vi "CreateTempSensorParam332.vi"(0 "Courbe Conv":string[](array[string]) caption="Courbe Conversion", 11 "Error in":errorcluster) -> (4 "Configurations":string[](array[string]), 6 "SavedOK":bool, 8 "ModèleSauv":i32, 15 "Error out":errorcluster)   [LabVIEW 2010]
doc: "Ce Vi sert à la création de modèles de configuration. À partir des différents paramètres d'entreés disponible, il crée une table qui constitue le modèle. Le VI permet la sauvegarde des nouveaux modèles et la gestion des modèles existant."
uses:
  <vilib>/Utility/error.llb/DialogType.ctl
  <vilib>/Utility/config.llb/NI_LVConfig.lvlib
panel:
  in  "SensorPar":T1={"TableTC"=0, "TableConv"=0, "Compensation"=1, "Type"=1} caption="Paramètre de configuration d'entrée" {"Compensation" items=["Off", "On"]; "Type" items=["Silicon Diode", "GaAlAs Diode", "Platinum 100 (250 Ohms)", "Platinum 100 (500 Ohms)", "Platinum 1000 Ohms", "NTC RTD 75mV 7.5 KOhms", "Thermocouple 25mV", "Thermocouple 50mV", "NTC RTD 75mV 75 Ohms", "NTC RTD 75mV 750 Ohms", "NTC RTD 75mV 7.5 KOhms", "NTC RTD 75mV 75 KOhms", "NTC RTD 75mV Auto"]; "TableTC" max=41 step=1}
  in  "Nom":string
  in  "Input":u8(ring)=3 caption="Entrées" items=["A", "B", "C", "D"]
  in  "OK":bool
  in  "Save":bool
  in  "Modèles":i32(listbox) caption="Modèles de \nConfiguration"
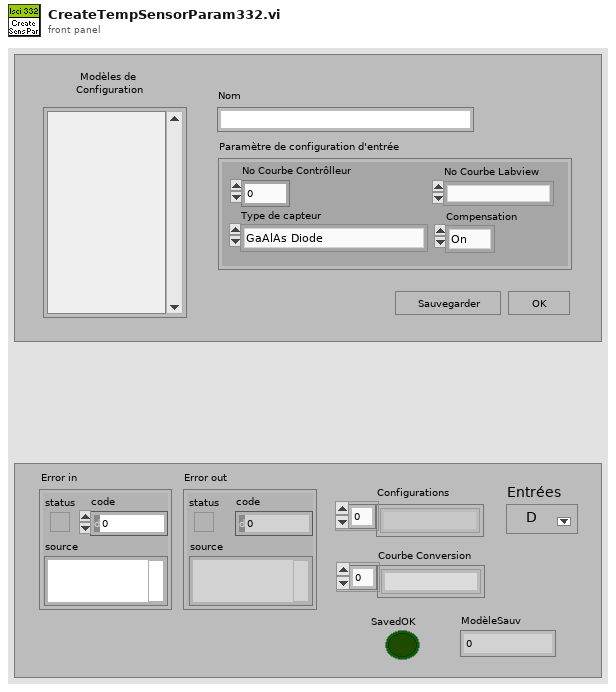
[diagram p1: front panel]
types:
  T1 = cluster{"TableTC":u16, "TableConv":u16, "Compensation":u16, "Type":u16}
  T2 = enum32{"Invalid", "Standard", "Closed", "Hidden", "Minimized", "Maximized"}
  T3 = typedef "InConfigPar332.ctl" = cluster{"TableTC":u16, "TableConv":u16, "Compensation":u16, "Type":u16}
  T4 = typedef "DialogType.ctl" = u16
  T5 = typedef "NI_LVConfig.lvlib/Config Data RefNum.ctl" = refnum<k1>
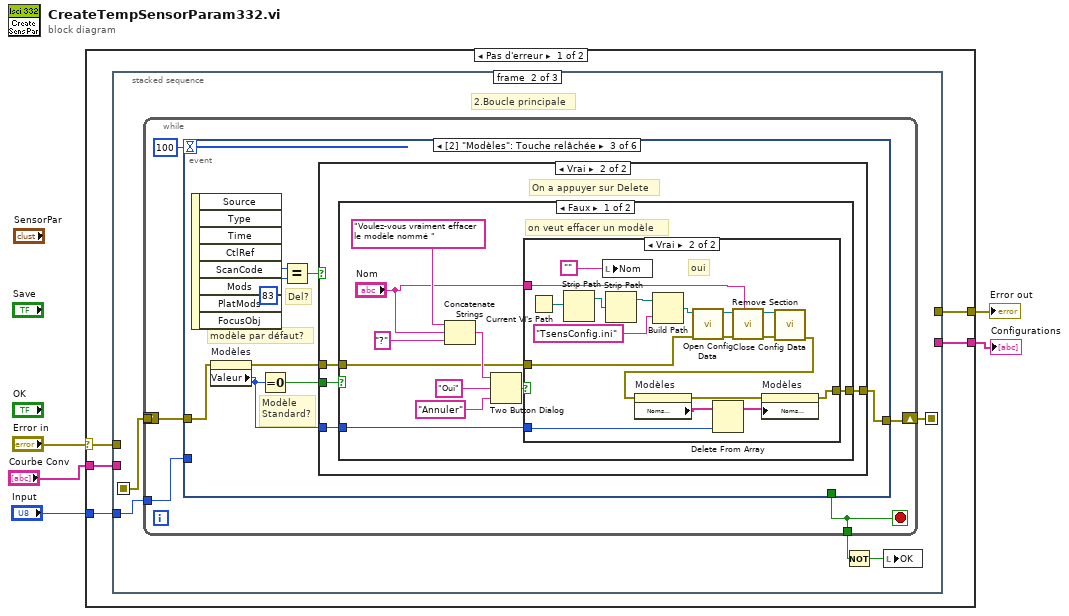
[diagram p0: block diagram]
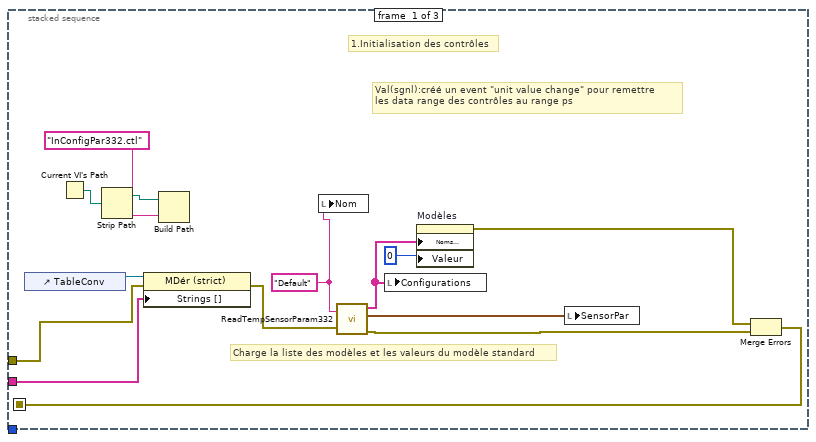
[diagram p2: hidden frame]
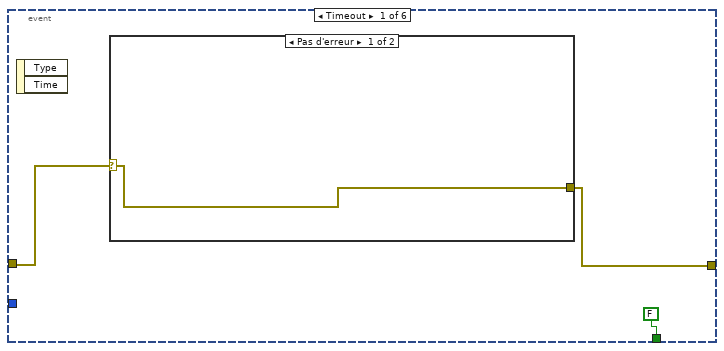
[diagram p3: hidden frame]
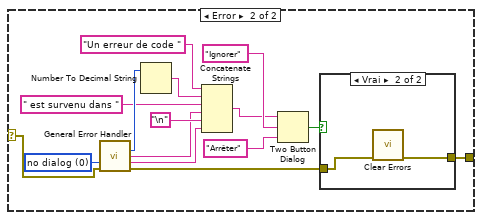
[diagram p4: hidden frame]
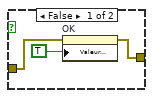
[diagram p5: hidden frame]
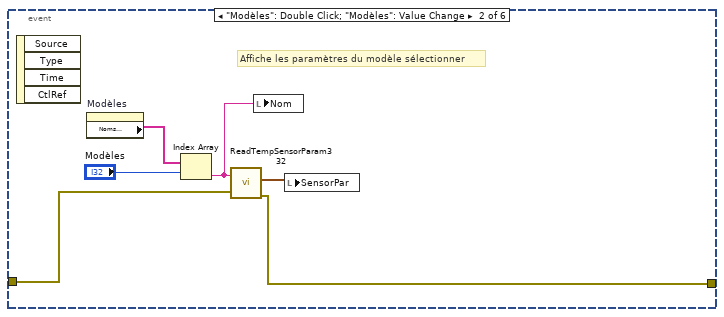
[diagram p6: hidden frame]
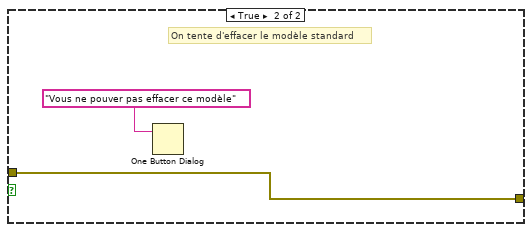
[diagram p9: hidden frame]
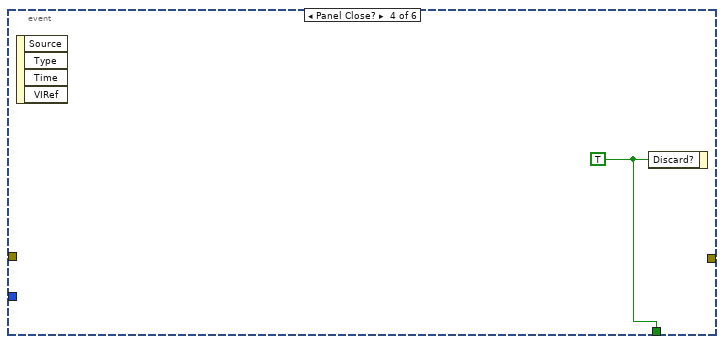
[diagram p10: hidden frame]
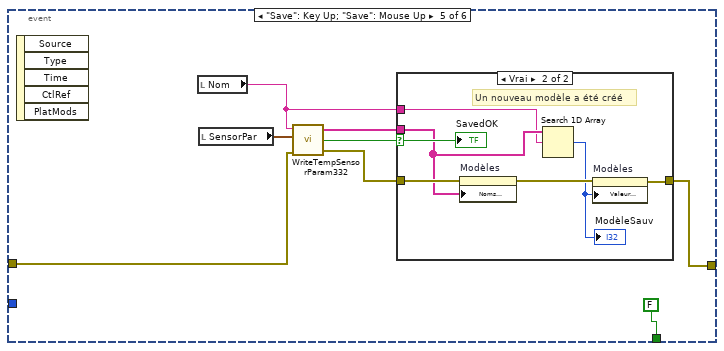
[diagram p11: hidden frame]
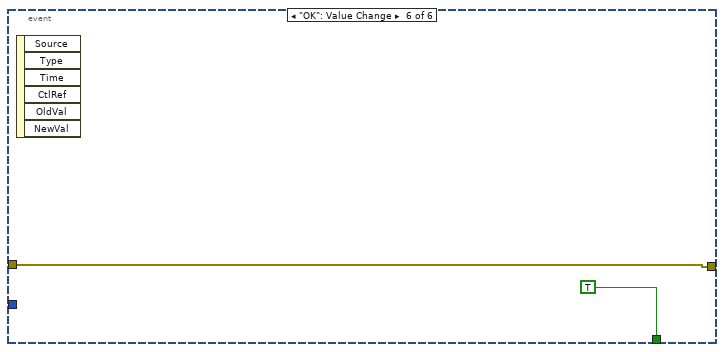
[diagram p13: hidden frame]
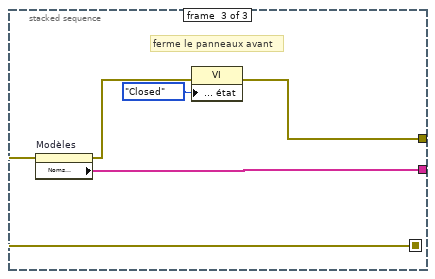
[diagram p14: hidden frame]
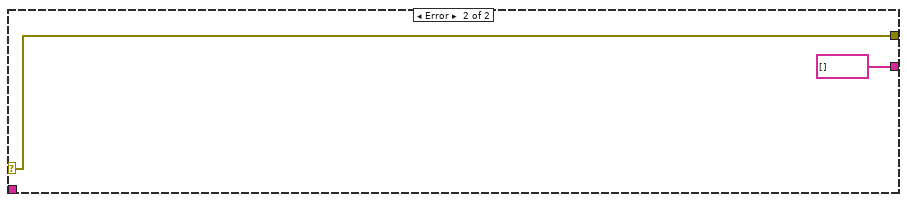
[diagram p15: hidden frame]
diagram:
  n1 = case shown="Pas d'erreur" "Error in" {
    selector: "Error in" -> [w10 w134]
    tunnel: [w8 w134] -> w5
    tunnel: [w9 string[] [] ("Item Names")] -> w2
    tunnel: "Input" -> [w7 _]
    tunnel: "Courbe Conv" -> [w6 _]
    frame No Error {
      n2 = stacked-sequence {
        seq-local: [w24 _ _] -> [_ w29 _]
        seq-local: [_ w28 _] -> [_ _ w131]
        tunnel: w10 -> [w13 _ _]
        tunnel: [_ _ w132] -> w9
        tunnel: [_ _ w128] -> w8
        tunnel: w7 -> [_ w25 _]
        tunnel: w6 -> [w11 _ _]
        frame #0 {
          w19 = "Default" ("Modèle")
          # "Val(sgnl):créé un event \"unit value change\" pour remettre \nles data range des contrôles au range ps"
          # "Charge la liste des modèles et les valeurs du modèle standard"
          # "1.Initialisation des contrôles"
          n3 = control-ref of="TableConv"() -> (w14:refnum<vi>)
          n4 = Current VI's Path() -> (path=w17:path)
          n5 = Strip Path(path=w17) -> (stripped path=w16:path)  [unwired: 1 out]
          n6 = property class="MDér (strict)"(reference=w14, error in=w13, "Strings []"=w11) -> (error out=w12:errorcluster)  [unwired: 1 out]
          n7 = Build Path(base path=w16, name or relative path="InConfigPar332.ctl" ("nom ou chemin relatif")) -> ()  [unwired: 1 out]
          n8 = local write "Nom"(w19) -> ()
          n9 = call <userlib>:"ReadTempSensorParam332.vi"("Nom"=w19, "Error in"=w12) -> ("Configurations"=w20:string[], "SensorPar"=w21:T3, "Error out"=w18:errorcluster)  [unwired: 1 in]
          n10 = local write "Configurations"(w20) -> ()
          n11 = property on="Modèles" class="LstDér (strict)"("Noms d'éléments"=w20, "Valeur"=0 ("Modèles")) -> (error out=w22:errorcluster)  [unwired: 2 in, 1 out]
          n12 = local write "SensorPar"(w21) -> ()
          n13 = Merge Errors(w22, w18) -> (w24:errorcluster)
        }
        frame #1 {
          # "2.Boucle principale"
          n14 = while {
            shift-right: [w33] -> w28
            shift-left: w29 -> [w32]
            tunnel: w29 -> [_]
            tunnel: [w31] -> w27
            tunnel: w25 -> [w30]
            stop <- w31 stop-if-true
            n15 = event shown="[2] \"Modèles\": Touche relâchée" {
              selector: _ -> [_ _ _ _ _ _]
              dyn-events: _ -> [_ _ _ _ _ _]
              timeout: 100 -> [_ _ _ _ _ _]
              tunnel: [FALSE ("status") _ _ w109 FALSE ("status") TRUE] -> w31
              tunnel: [w36 w63 w66 _ w114 w126] -> w33
              tunnel: w32 -> [w35 w62 w68 _ w116 w126]
              tunnel: w30 -> [_ _ _ _ _ _]
              event Timeout {
                n16 = event-data() -> ()  [unwired: 1 in, 2 out]
                n17 = case shown="Pas d'erreur" w35 {
                  selector: w35 -> [w38 w39]
                  tunnel: [w38 w40] -> w36
                  frame No Error {
                  }
                  frame Error {
                    w50 = T4 0 items=["no dialog", "OK message", "continue or stop message", "OK message + warnings", "continue/stop + warnings"] ("type of dialog (OK msg:1)")
                    n18 = call <vilib>:"General Error Handler.vi"("type of dialog (OK msg:1)"=w50, "error in (no error)"=w39) -> ("code out"=w46:i32, "source out"=w45:string, "message"=w43:string, "error out"=w41:errorcluster)  [unwired: 9 in, 1 out]
                    n19 = Number To Decimal String(number=w46) -> (decimal integer string=w47:string)  [unwired: 1 in]
                    n20 = Concatenate Strings("Un erreur de code " ("string"), w47, " est survenu dans " ("string"), w45, "\n", w43) -> (w42:string)
                    n21 = Two Button Dialog(message=w42, 1:"Arrêter" ("F button name (\"Cancel\")"), 2:"Ignorer" ("T button name (\"OK\")")) -> (T button?=w53:bool)
                    n22 = case shown="Vrai" w53 {
                      tunnel: w41 -> [w55 w58]
                      tunnel: [w54 w57] -> w40
                      frame False {
                        n23 = property on="OK" class="Bool (strict)"(error in=w55, "Valeur (Signalisation)"=TRUE ("Value (Signaling)")) -> (error out=w54:errorcluster)  [unwired: 1 in, 1 out]
                      }
                      frame True {
                        n24 = call <vilib>:"Clear Errors.vi"("error in (no error)"=w58) -> ("error out"=w57:errorcluster)  [unwired: 6 in]
                      }
                    }
                  }
                }
              }
              event "Modèles": Double Click; "Modèles": Value Change {
                # "Affiche les paramètres du modèle sélectionner"
                n25 = event-data() -> ()  [unwired: 1 in, 4 out]
                n26 = property on="Modèles" class="LstDér (strict)"() -> ("Noms d'éléments"=w60:string[])  [unwired: 2 in, 2 out]
                n27 = Index Array(array=w60, index="Modèles") -> (element=w64:string)
                n28 = call <userlib>:"ReadTempSensorParam332.vi"("Nom"=w64, "Error in"=w62) -> ("SensorPar"=w59:T3, "Error out"=w63:errorcluster)  [unwired: 1 in, 1 out]
                n29 = local write "Nom"(w64) -> ()
                n30 = local write "SensorPar"(w59) -> ()
              }
              event "Modèles": Key Up {
                # "Modèle\nStandard?"
                # "Del?"
                # "modèle par défaut?"
                n31 = event-data() -> ("ScanCode"=w72:i16)  [unwired: 1 in, 7 out]
                n32 = property on="Modèles" class="LstDér (strict)"(error in=w68) -> (error out=w67:errorcluster, "Valeur"=w69:i32)  [unwired: 1 in, 1 out]
                n33 = Equal To 0?(x=w69) -> (x = 0?=w70:bool)
                n34 = Equal?(x=w72, y=i16 83) -> (x = y?=w71:bool)
                n35 = case shown="Vrai" w71 {
                  tunnel: w70 -> [_ w77]
                  tunnel: w69 -> [_ w76]
                  tunnel: w67 -> [w73 w75]
                  tunnel: [w73 w74] -> w66
                  frame False {
                  }
                  frame True {
                    # "On a appuyer sur Delete"
                    n36 = case shown="Faux" w77 {
                      tunnel: w76 -> [w81 _]
                      tunnel: w75 -> [w80 w107]
                      tunnel: [w79 w107] -> w74
                      frame False {
                        # "on veut effacer un modèle"
                        n37 = Concatenate Strings("Voulez-vous vraiment effacer le modèle nommé " ("string"), "Nom", "?" ("string")) -> (w85:string)
                        n38 = Two Button Dialog(message=w85, 1:"Annuler" ("T button name (\"OK\")"), 2:"Oui" ("T button name (\"OK\")")) -> (T button?=w82:bool)
                        n39 = case shown="Vrai" w82 {
                          tunnel: w81 -> [_ w94]
                          tunnel: w80 -> [w88 w98]
                          tunnel: [w88 w95] -> w79
                          tunnel: "Nom" -> [_ w92]
                          frame False {
                            # "non"
                          }
                          frame True {
                            # "oui"
                            n40 = Current VI's Path() -> (path=w104:path)
                            n41 = Strip Path(path=w104) -> (stripped path=w89:path)  [unwired: 1 out]
                            n42 = local write "Nom"("") -> ()
                            n43 = Strip Path(path=w89) -> (stripped path=w90:path)  [unwired: 1 out]
                            n44 = Build Path(base path=w90, name or relative path="TsensConfig.ini") -> (appended path=w106:path)
                            n45 = call <vilib>:"Open Config Data.vi"("error in (no error)"=w98, "configuration file path"=w106) -> ("error out"=w103:errorcluster, "refnum"=w102:T5)  [unwired: 7 in, 1 out]
                            n46 = call <vilib>:"Remove Section.vi"("section"=w92, "error in (no error)"=w103, "refnum"=w102) -> ("error out"=w100:errorcluster, "refnum out"=w101:T5)  [unwired: 6 in, 1 out]
                            n47 = call <vilib>:"Close Config Data.vi"("error in (no error)"=w100, "refnum"=w101) -> ("error out"=w96:errorcluster)  [unwired: 8 in, 1 out]
                            n48 = property on="Modèles" class="LstDér (strict)"(error in=w96) -> (error out=w97:errorcluster, "Noms d'éléments"=w99:string[])  [unwired: 1 in, 1 out]
                            n49 = Delete From Array(array=w99, index=w94) -> (array with subset deleted=w93:string[])  [unwired: 1 in, 1 out]
                            n50 = property on="Modèles" class="LstDér (strict)"(error in=w97, "Noms d'éléments"=w93) -> (error out=w95:errorcluster)  [unwired: 1 in, 1 out]
                          }
                        }
                      }
                      frame True {
                        # "On tente d'effacer le modèle standard"
                        n51 = One Button Dialog(message="Vous ne pouver pas effacer ce modèle") -> ()  [unwired: 1 in, 1 out]
                      }
                    }
                  }
                }
              }
              event Panel Close? {
                w109 = TRUE
                n52 = event-data() -> ()  [unwired: 1 in, 4 out]
                n53 = event-data("Discard?"=w109) -> ()  [unwired: 1 in, 1 out]
              }
              event "Save": Key Up; "Save": Mouse Up {
                n54 = event-data() -> ()  [unwired: 1 in, 5 out]
                n55 = local read "Nom"() -> (w110:string)
                n56 = local read "SensorPar"() -> (w111:T1)
                n57 = call <userlib>:"WriteTempSensorParam332.vi"("Error in"=w116, "SensorPar"=w111, "Nom"=w110) -> ("Error out"=w115:errorcluster, "SavedOK"=w117:bool, "Configurations"=w113:string[])  [unwired: 1 in]
                n58 = case shown="Vrai" w117 {
                  selector: w117 -> [_ w124]
                  tunnel: [w118 w122] -> w114
                  tunnel: w115 -> [w118 w125]
                  tunnel: w113 -> [_ w121]
                  tunnel: w110 -> [_ w119]
                  frame False {
                    # "La création n'a pas eu lieu"
                  }
                  frame True {
                    # "Un nouveau modèle a été créé"
                    n59 = property on="Modèles" class="LstDér (strict)"(error in=w125, "Noms d'éléments"=w121) -> (error out=w123:errorcluster)  [unwired: 1 in, 1 out]
                    n60 = Search 1D Array(1D array=w121, element=w119) -> (index of element=w120:i32)  [unwired: 1 in]
                    "ModèleSauv" <- w120
                    n61 = property on="Modèles" class="LstDér (strict)"(error in=w123, "Valeur (Signalisation)"=w120) -> (error out=w122:errorcluster)  [unwired: 1 in, 1 out]
                    "SavedOK" <- w124
                  }
                }
              }
              event "OK": Value Change {
                n62 = event-data() -> ()  [unwired: 1 in, 6 out]
              }
            }
          }
          n63 = Not(x=w27) -> (.not. x?=w26:bool)
          n64 = local write "OK"(w26) -> ()
        }
        frame #2 {
          # "ferme le panneaux avant"
          n65 = property on="Modèles" class="LstDér (strict)"(error in=w131) -> (error out=w130:errorcluster, "Noms d'éléments"=w132:string[])  [unwired: 1 in, 1 out]
          n66 = property class="VI"(error in=w130, "Fenêtre face-avant : état"=T2."Closed" ("Front Panel Window:State")) -> (error out=w128:errorcluster)  [unwired: 1 in, 1 out]
        }
      }
    }
    frame Error {
    }
  }
  "Error out" <- w5
  "Configurations" <- w2
